vi "Dialog Window Time Out.vi"(6 "Front Panel Window:Panel Bounds":T1, 7 "Üzenet be":string, 8 "Error In":errorcluster) -> (0 "Error Out":errorcluster)   [LabVIEW 2014]
uses:
  <vilib>/Utility/miscctls.llb/LVRectTypeDef.ctl
panel:
  out "Üzenet":string
  in  "Time Out":bool
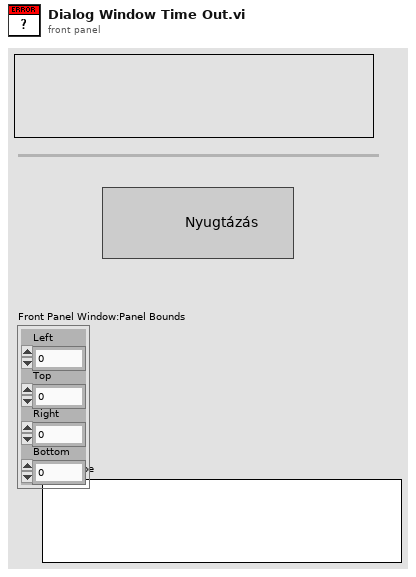
[diagram p1: front panel]
types:
  T1 = typedef "LVRectTypeDef.ctl" = cluster{"Left":i16, "Top":i16, "Right":i16, "Bottom":i16}
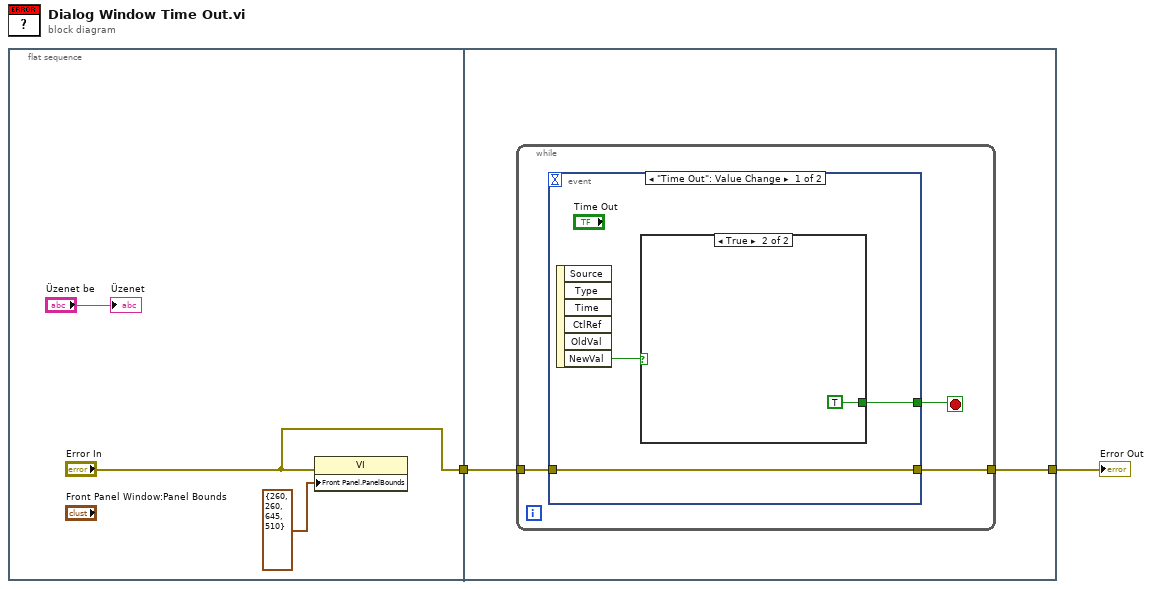
[diagram p0: block diagram]
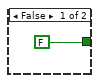
[diagram p2: hidden frame]
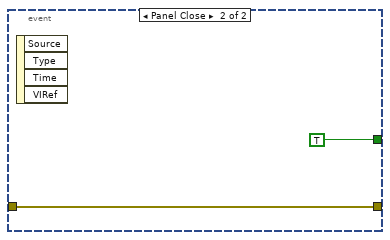
[diagram p3: hidden frame]
diagram:
  n1 = flat-sequence {
    tunnel: ["Error In"] -> w1
    tunnel: w1 -> [w7]
    tunnel: [w6] -> w2
    frame #0 {
      n2 = property class="VI"(error in="Error In", "Front Panel.PanelBounds"=T1 {"Left"=260, "Top"=260, "Right"=645, "Bottom"=510} ("Front Panel Window:Panel Bounds")) -> ()  [unwired: 1 in, 2 out]
      "Üzenet" <- "Üzenet be"
    }
    frame #1 {
      n3 = while {
        tunnel: w7 -> [w10]
        tunnel: [w9] -> w6
        stop <- w8 stop-if-true
        n4 = event shown="[0] \"Time Out\": Value Change" {
          selector: _ -> [_ _]
          dyn-events: _ -> [_ _]
          timeout: _ -> [_ _]
          tunnel: [w13 w17] -> w9
          tunnel: w10 -> [w13 w17]
          tunnel: [w11 TRUE] -> w8
          event "Time Out": Value Change {
            n5 = event-data() -> ("NewVal"=w12:bool)  [unwired: 1 in, 5 out]
            n6 = case shown="True" w12 {
              tunnel: [FALSE TRUE] -> w11
              frame False {
              }
              frame True {
              }
            }
          }
          event Panel Close {
            n7 = event-data() -> ()  [unwired: 1 in, 4 out]
          }
        }
      }
    }
  }
  "Error Out" <- w2
